vi "Transfer Images Data to UI - Copy.vi"(0 "fpga interface in":refnum<k20>, 1 "'stop' notifier":refnum<notifier>, 2 "queue out":refnum<queue>, 3 "measure call context in":refnum<class "Measure Call Context.lvclass">, 7 "display channel number":i32, 11 "error in":errorcluster, 13 "raw display notifier":refnum<notifier>) -> (4 "fpga interface out":refnum<k20>, 15 "error out":errorcluster)   [LabVIEW 2025, in "Automotive Vision.lvclass"]
doc: "Handles frame grabbing, and prepare data for sendig it to the UI."
uses:
  Automotive Vision.lvclass
  <vilib>/Plug-In SDKs/Measurements/Measure Call Context/Measure Call Context.lvclass
  <vilib>/rvi/interface/nirviReadWriteControl/nirviReadWriteControl.xnode
  Automotive Vision.lvclass/Automotive Vision.ctl
  deps/NI148X/Getting Started/Host/Common/GettingStarted_Common_148X_Host.lvlib
  deps/NI148X/Getting Started/Host/Common/Types/148x_Common_FPGA_Reference.ctl
  <instrlib>/FlexRIO/CSI-2/v2/Common/Types/LLP Data Type.ctl
  <instrlib>/FlexRIO/CSI-2/v2/Common/NI CSI-2 API Common v2.lvlib
  Automotive-Vision OOB Data Transfer/Automotive-Vision OOB Data Transfer.lvlib
  Measurement Results.ctl
  NiFpgaLv.dll
  <vilib>/Utility/error.llb/Error Cluster From Error Code.vi
  <vilib>/rvi/interface/Simulation/niFpgaSimulationCallBeginRW.vi
  <vilib>/rvi/errors/niLvFpgaAdjustHostInterfaceError.vi
  <vilib>/vision/Image Controls.llb/IMAQ Image.ctl
  deps/NI148X/Getting Started/Host/Common/Types/RAW Interpretation for Display.ctl
  deps/NI148X/Getting Started/Host/Common/Types/Serial Channel Display Parameters.ctl
  Status Data.ctl
  Image Info.ctl
panel:
  in  "Image Info":T1
  out "Image Pixels (U32)":u32[](array[numeric])
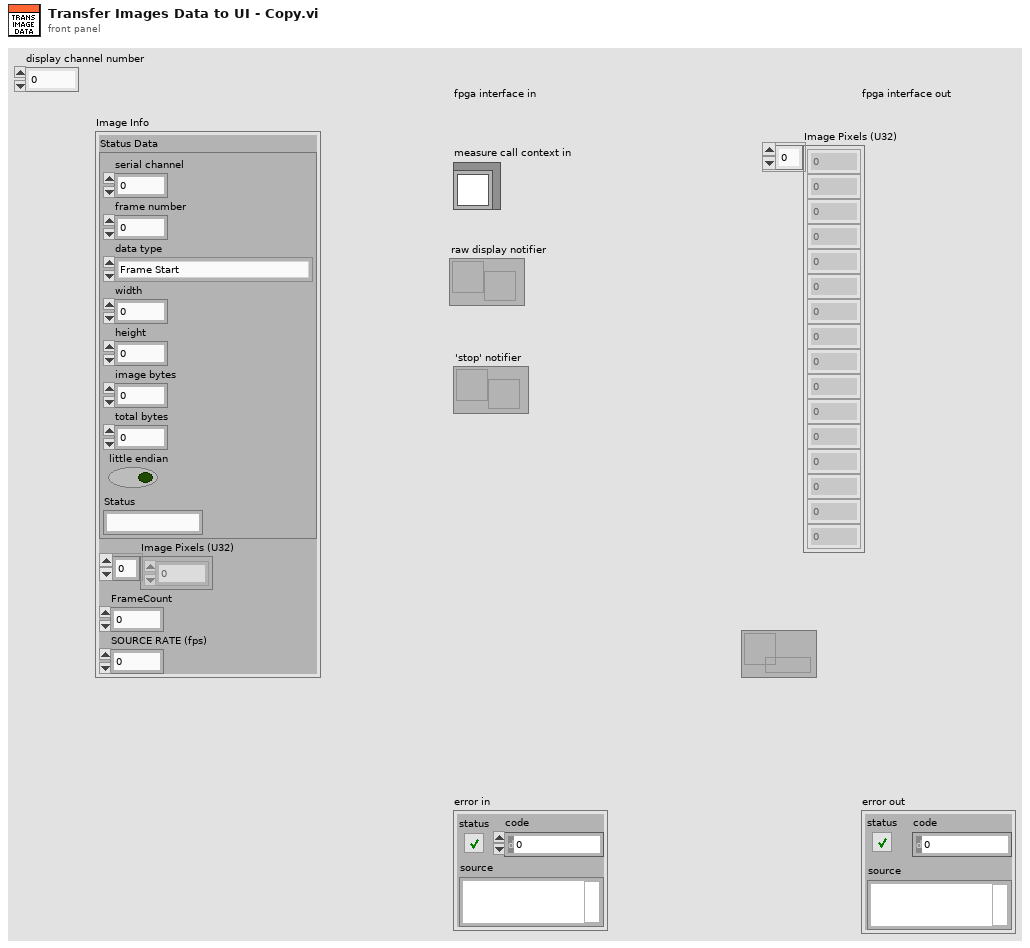
[diagram p1: front panel]
types:
  T1 = typedef "Image Info.ctl" = cluster{"Status Data":T2, "Image Pixels (U32)":u32[], "FrameCount":u64, "SOURCE RATE (fps)":dbl}
  T2 = typedef "Status Data.ctl" = cluster{"serial channel":fxp<+,3,3>, "frame number":u16, "data type":T3, "width":u16, "height":u16, "image bytes":u32, "total bytes":u32, "little endian":bool, "Status":string}
  T3 = typedef "NI CSI-2 API Common v2.lvlib/LLP Data Type.ctl" = enum8{"Frame Start", "Frame End", "Line Start", "Line End", "End of Transmission", "Reserved 0", "Reserved 1", "Reserved 2", "Generic Short Packet 1", "Generic Short Packet 2", "Generic Short Packet 3", "Generic Short Packet 4", "Generic Short Packet 5", "Generic Short Packet 6", "Generic Short Packet 7", "Generic Short Packet 8", "Null", "Blanking Data", "Embedded 8-bit non Image Data", "Generic Long Packet 1", "Generic Long Packet 2", "Generic Long Packet 3", "Generic Long Packet 4", "Reserved 3", "YUV420 8-bit", "YUV420 10-bit", "Legacy YUV420 8-bit", "Reserved 4", "YUV420 8-bit Chroma Shifted", "YUV420 10-bit Chroma Shifted", "YUV422 8-bit", "YUV422 10-bit", "RGB444", "RGB555", "RGB565", "RGB666", "RGB888", "Reserved 5", "Reserved 6", "RAW 24", "RAW 6", "RAW 7", "RAW 8", "RAW 10", "RAW 12", "RAW 14", "RAW 16", "RAW 20", "User Defined 8-bit Data 1", "User Defined 8-bit Data 2", "User Defined 8-bit Data 3", "User Defined 8-bit Data 4", "User Defined 8-bit Data 5", "User Defined 8-bit Data 6", "User Defined 8-bit Data 7", "User Defined 8-bit Data 8", "USL Command", "Reserved 7", "Reserved 8", "Reserved 9", "Reserved 10", "Reserved 11", "Reserved 12", "LRTE EPD Spacer"}
  T4 = cluster{"serial channel":fxp<+,3,3>, "frame number":u16, "data type":T3, "width":u16, "height":u16, "image bytes":u32, "total bytes":u32, "little endian":bool, "Status":string}
  T5 = typedef "GettingStarted_Common_148X_Host.lvlib/148x_Common_FPGA_Reference.ctl" = refnum<k20>
  T6 = typedef "GettingStarted_Common_148X_Host.lvlib/Serial Channel Display Parameters.ctl" = cluster{"images":cluster{"grayscale":T7, "color":T7}, "RAW parameters":cluster{"interpretation":T8, "bayer parameters":cluster{"pattern":i32, "algorithm":i32, "red gain":dbl, "green gain":dbl, "blue gain":dbl}}}
  T7 = typedef "IMAQ Image.ctl" = refnum<image>
  T8 = typedef "GettingStarted_Common_148X_Host.lvlib/RAW Interpretation for Display.ctl" = enum16{"Grayscale", "Bayer", "RGB", "YUV422", "YUV420", "Legacy YUV420"}
  T9 = typedef "GettingStarted_Common_148X_FPGA.lvlib/Image Metadata.ctl" = cluster{"serial channel":fxp<+,3,3>, "frame number":u16, "data type":T3, "width":u16, "height":u16, "image bytes":u32, "total bytes":u32, "little endian":bool}
  T10 = typedef "Automotive-Vision OOB Data Transfer.lvlib/OOB to Logic Data.ctl" = cluster{"PauseResume":bool, "ExportPath":string, "ExportType":u16, "Export":bool}
  T11 = typedef "Automotive Vision.lvclass/Measurement Results.ctl" = cluster{"ACQ. IN PROGRESS":bool, "IMAGE PIXEL DATA":u32[], "ACQ. DURATION (s)":dbl, "SOURCE RATE (fps)":dbl, "BYTES ACQUIRED":u64, "FRAME COUNT":u64, "POC VOLTAGE (V)":dbl, "POC CURRENT (A)":dbl, "ERROR":bool, "STATE MESSAGE":string, "IMAGE DATA":string, "OOB gRPC Port":i32, "HEIGHT":u64, "WIDTH":u64, "IMAGE SIZE":u64}
  T12 = cluster{"image pixel data fifo overflow":bool, "image metadata fifo overflow":bool}[]
  T13 = cluster{"image pixel data fifo overflow":bool, "image metadata fifo overflow":bool}
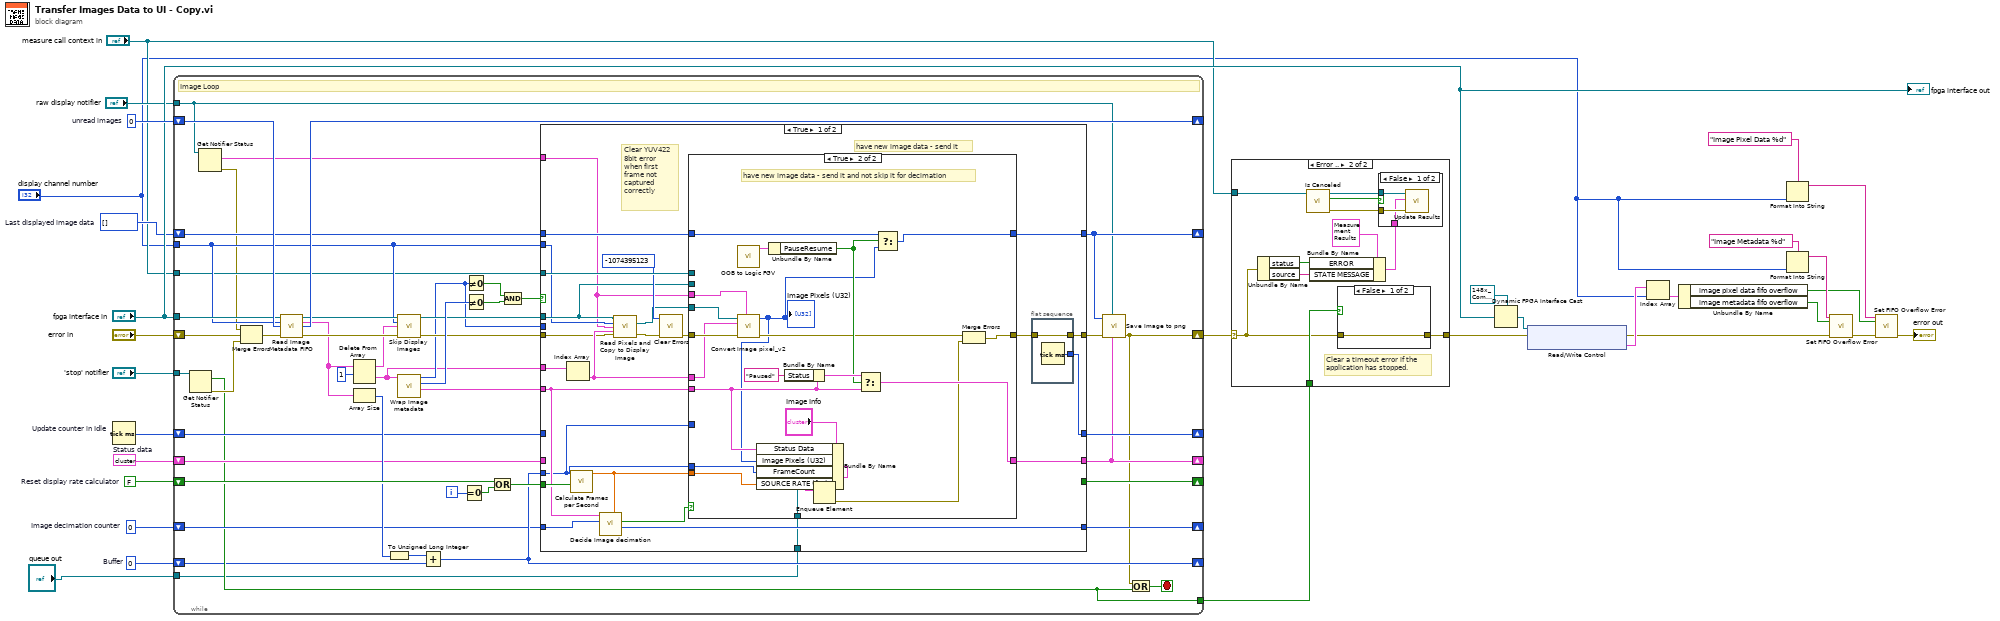
[diagram p0: block diagram]
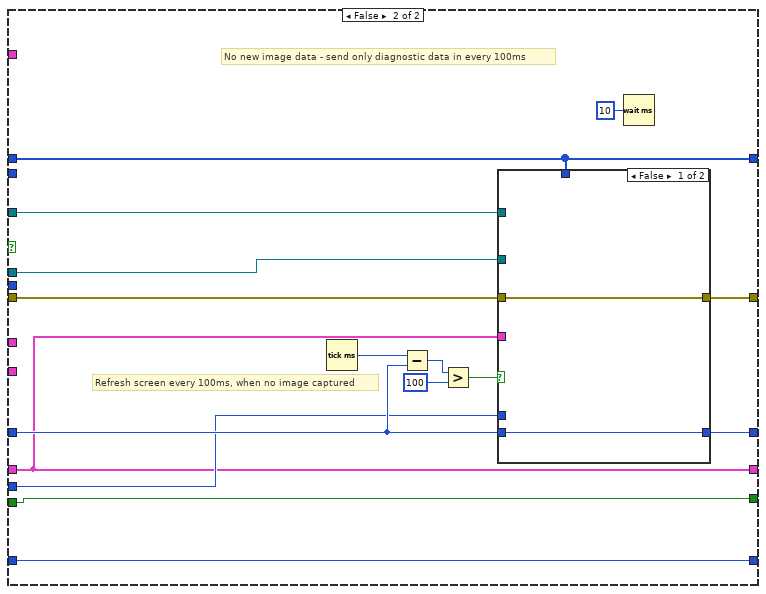
[diagram p3: hidden frame]
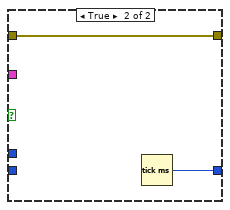
[diagram p4: hidden frame]
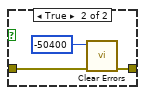
[diagram p7: hidden frame]
diagram:
  w5 = T4 {"serial channel"=0.0, "frame number"=0, "data type"=enum."Frame Start", "width"=0, "height"=0, "image bytes"=0, "total bytes"=0, "little endian"=FALSE, "Status"="Ready for Acquisition"}  # Status data
  w7 = u32 0  # Image decimation counter
  w8 = u32[] []  # Last displayed image data
  w14 = u32 0  # Buffer
  w15 = FALSE  # Reset display rate calculator
  w30 = u32 0  # unread images
  n1 = Tick Count (ms) "Update counter in Idle"() -> (millisecond timer value=w9:u32)
  n2 = while {
    shift-right: [w36] -> w13
    shift-left: "error in" -> [w53]
    tunnel: "fpga interface in" -> [w56]
    shift-right: [w76] -> _
    shift-left: w30 -> [w67]
    tunnel: "display channel number" -> [w52]
    shift-right: [w71] -> _
    shift-left: w15 -> [w68]
    shift-right: [w58] -> _
    shift-left: w14 -> [w40]
    tunnel: [w42] -> w11
    tunnel: "'stop' notifier" -> [w55]
    shift-right: [w50] -> _
    shift-left: w9 -> [w51]
    shift-right: [w39] -> _
    shift-left: w8 -> [w49]
    shift-right: [w47] -> _
    shift-left: w7 -> [w48]
    tunnel: "measure call context in" -> [w46]
    shift-right: [w37] -> _
    shift-left: w5 -> [w45]
    tunnel: "raw display notifier" -> [w35]
    tunnel: "queue out" -> [w31]
    i -> [w75]
    stop <- w77 stop-if-true
    # "Image Loop"
    n3 = Get Notifier Status(notifier=w55) -> (current notification=w42:bool, error out=w78:errorcluster)  [unwired: 1 in, 3 out]
    n4 = Get Notifier Status(notifier=w35) -> (current notification=w33:T6[], error out=w34:errorcluster)  [unwired: 1 in, 3 out]
    n5 = Merge Errors(w34, w53, w78) -> (w54:errorcluster)
    n6 = call "Read Image Metadata FIFO.vi"("fpga inteface in"=w56, "display channel number"=w52, "number of images"=w67, "error in (no error)"=w54) -> ("fpga interface out"=w64:refnum<k20>, "image metadata"=w57:T9[], "images remaining"=w76:u32, "error out"=w61:errorcluster)  [unwired: 8 in]
    n7 = Delete From Array(array=w57, length=1) -> (deleted portion=w32:T9[], array with subset deleted=w60:T9[])  [unwired: 1 in]
    n8 = Array Size(array=w57) -> (size(s)=w59:i32)
    n9 = To Unsigned Long Integer(number=w59) -> (unsigned 32bit integer=w41:u32)
    n10 = call "Skip Display Images.vi"("fpga interface in"=w64, "display channel number"=w52, "image metadata"=w60, "error in (no error)"=w61) -> ("fpga interface out"=w63:refnum<k20>, "error out"=w62:errorcluster)  [unwired: 10 in]
    n11 = call "Wrap Image metadata.vi"("image metadata"=w32) -> ("element"=w44:T4, "Numeric"=w66:i32, "total bytes"=w43:u32)  [unwired: 8 in]
    n12 = Add(x=w41, y=w40) -> (x+y=w58:u32)
    n13 = Equal To 0?(x=w75) -> (x = 0?=w69:bool)
    n14 = Not Equal To 0?(x=w43) -> (x != 0?=w73:bool)
    n15 = Not Equal To 0?(x=w66) -> (x != 0?=w74:bool)
    n16 = Compound Arithmetic op=OR(w68, w69) -> (w70:bool)
    n17 = Compound Arithmetic op=AND(w73, w74) -> (w72:bool)
    n18 = case shown="True" w72 {
      tunnel: w62 -> [w81 w130]
      tunnel: w63 -> [w85 w129]
      tunnel: w52 -> [w84 _]
      tunnel: [w101 w137] -> w38
      tunnel: w70 -> [w93 w144]
      tunnel: [_ w144] -> w71
      tunnel: w58 -> [w79 w134]
      tunnel: w43 -> [_ _]
      tunnel: w44 -> [w90 _]
      tunnel: w46 -> [w102 w131]
      tunnel: w51 -> [_ w136]
      tunnel: [w100 w138] -> w50
      tunnel: w49 -> [w98 w135]
      tunnel: [w99 w135] -> w39
      tunnel: w48 -> [w97 w133]
      tunnel: [w96 w133] -> w47
      tunnel: w45 -> [_ w132]
      tunnel: [w94 w132] -> w37
      tunnel: w33 -> [w83 _]
      tunnel: w32 -> [w91 _]
      tunnel: w31 -> [w80 _]
      frame True {
        # "Clear YUV422 8bit error when first frame not captured correctly"
        # "have new image data - send it"
        n19 = Index Array(array=w91) -> (element=w82:T9)  [unwired: 1 in]
        n20 = call <vilib>:"Calculate Frames per Second.vi"("Reset"=w93, "Buffer Number"=w79) -> ("Acquired Frames/s"=w89:dbl)  [unwired: 7 in, 2 out]
        n21 = call "Decide Image decimation.vi"("FPS"=w89, "Image decimation counter in"=w97, "element in"=w90) -> ("Image decimation counter out"=w96:u32, "send current image data"=w95:bool)  [unwired: 7 in]
        n22 = call "Read Pixels and Copy to Display Image.vi"("fpga interface in"=w85, "display channel number"=w84, "serial channel display parameters"=w83, "image metadata"=w82) -> ("display image"=w86:T7)  [unwired: 9 in, 2 out]
        n23 = call <vilib>:"Clear Errors.vi"("error in (no error)"=w81, "specific error code to clear (0: all)"=-1074395123) -> ("error out"=w87:errorcluster)  [unwired: 4 in, 1 out]
        n24 = case shown="True" w95 {
          tunnel: [w103 w113] -> w92
          tunnel: w89 -> [_ w106]
          tunnel: w90 -> [w104 w110]
          tunnel: w102 -> [_ _]
          tunnel: [w105 w126] -> w99
          tunnel: w79 -> [_ _]
          tunnel: w98 -> [w105 w125]
          tunnel: [w104 w124] -> w94
          tunnel: w85 -> [_ _]
          tunnel: w87 -> [w103 w119]
          tunnel: w86 -> [_ w117]
          tunnel: w82 -> [_ w116]
          tunnel: w83 -> [_ w115]
          tunnel: w80 -> [_ w114]
          tunnel: w79 -> [_ w107]
          frame False {
            # "have new image data - but skip the sending to not overload UI with data transfer"
          }
          frame True {
            # "have new image data - send it and not skip it for decimation"
            n25 = call "OOB to Logic FGV.vi"() -> ("OOB to Logic Data out"=w121:T10)  [unwired: 10 in, 1 out]
            n26 = call "Convert Image pixel_v2.vi"("serial channel display parameters"=w115, "error in"=w119, "image metadata"=w116, "Refnum in"=w117) -> ("error out"=w118:errorcluster, "Image Pixels (U32)"=w109:u32[])  [unwired: 6 in]
            "Image Pixels (U32)" <- w109
            n27 = Bundle By Name(cluster="Image Info", "Status Data"=w110, "Image Pixels (U32)"=w109, "FrameCount"=w107, "SOURCE RATE (fps)"=w106) -> (w108:T1)
            n28 = Unbundle By Name(w121) -> ("PauseResume"=w120:bool)
            n29 = Bundle By Name(cluster=w110, "Status"="Paused") -> (w123:T4)
            n30 = Enqueue Element(queue=w114, element=w108) -> (error out=w112:errorcluster)  [unwired: 2 in, 2 out]
            n31 = Select(t=w123, s=w120, f=w110) -> (s? t:f=w124:T4)
            n32 = Select(t=w125, s=w120, f=w109) -> (s? t:f=w126:u32[])
            n33 = Merge Errors(w118, w112) -> (w113:errorcluster)
          }
        }
        n34 = flat-sequence {
          tunnel: [w128] -> w101
          tunnel: w92 -> [w128]
          tunnel: [w127] -> w100
          frame #0 {
            n35 = Tick Count (ms)() -> (millisecond timer value=w127:u32)
          }
        }
      }
      frame False {
        # "Refresh screen every 100ms, when no image captured"
        # "No new image data - send only diagnostic data in every 100ms"
        n36 = Tick Count (ms)() -> (millisecond timer value=w142:u32)
        n37 = Subtract(x=w142, y=w136) -> (x-y=w141:u32)
        n38 = Greater?(x=w141, y=u32 100) -> (0:w139:bool)
        n39 = case shown="False" w139 {
          tunnel: w130 -> [w146 w147]
          tunnel: [w146 w147] -> w137
          tunnel: w132 -> [_ _]
          tunnel: [w145 w148] -> w138
          tunnel: w136 -> [w145 _]
          tunnel: w135 -> [_ _]
          tunnel: w134 -> [_ _]
          tunnel: w131 -> [_ _]
          tunnel: w129 -> [_ _]
          frame False {
          }
          frame True {
            n40 = Tick Count (ms)() -> (millisecond timer value=w148:u32)
          }
        }
        n41 = Wait (ms)(milliseconds to wait=u32 10) -> ()  [unwired: 1 out]
      }
    }
    n42 = call "Save Image to png.vi"("image metadata"=w37, "raw display notifier"=w35, "error in"=w38, "Last displayed image data"=w39) -> ("error out"=w36:errorcluster)  [unwired: 7 in]
    n43 = Compound Arithmetic op=OR(w36, w42) -> (w77:bool)
  }
  n44 = case shown="Error .." w13 {
    selector: w13 -> [w149 w153]
    tunnel: [w149 w160] -> w25
    tunnel: w11 -> [_ w159]
    tunnel: "measure call context in" -> [_ w150]
    frame No Error {
    }
    frame Error {
      # "Clear a timeout error if the application has stopped."
      n45 = Unbundle By Name(w153) -> ("status"=w152:bool, "source"=w151:string)
      n46 = call <vilib>:"Is Canceled.vi"("measure call context in"=w150) -> ("error out"=w157:errorcluster, "is canceled?"=w156:bool, "measure call context out"=w158:refnum<class "Measure Call Context.lvclass">)  [unwired: 8 in]
      n47 = Bundle By Name(cluster=T11 {"ACQ. IN PROGRESS"=FALSE, "IMAGE PIXEL DATA"=[], "ACQ. DURATION (s)"=0.0, "SOURCE RATE (fps)"=0.0, "BYTES ACQUIRED"=0, "FRAME COUNT"=0, "POC VOLTAGE (V)"=0.0, "POC CURRENT (A)"=0.0, "ERROR"=FALSE, "STATE MESSAGE"="", "IMAGE DATA"="", "OOB gRPC Port"=0, "HEIGHT"=0, "WIDTH"=0, "IMAGE SIZE"=0} ("Measurement Results"), "ERROR"=w152, "STATE MESSAGE"=w151) -> (w154:T11)
      n48 = case shown="False" w159 {
        tunnel: w153 -> [w164 w167]
        tunnel: [w164 w165] -> w160
        frame False {
        }
        frame True {
          n49 = call <vilib>:"Clear Errors.vi"("error in (no error)"=w167, "specific error code to clear (0: all)"=-50400 ("y")) -> ("error out"=w165:errorcluster)  [unwired: 4 in, 1 out]
        }
      }
      n50 = case shown="False" w156 {
        tunnel: w158 -> [w163 _]
        tunnel: w157 -> [w162 _]
        tunnel: w154 -> [w161 _]
        frame False {
          n51 = call <vilib>:"Update Results.vi"("error in"=w162, "measurement results"=w161, "measure call context in"=w163) -> ()  [unwired: 7 in, 2 out]
        }
        frame True {
        }
      }
    }
  }
  n52 = Dynamic FPGA Interface Cast(Session In=T5 refnum ("FPGA VI Reference Out"), Type="fpga interface in") -> (Session Out=w26:T5)
  n53 = xnode ("Read/Write Control")("FPGA VI Reference In"=w26, "error in"=w25) -> ("error out"=w24:errorcluster, "display channel status"=w28:T12)  [unwired: 1 out]
  n54 = Index Array(array=w28, index="display channel number") -> (element=w29:T13)
  n55 = Unbundle By Name(w29) -> ("image pixel data fifo overflow"=w17:bool, "image metadata fifo overflow"=w16:bool)
  n56 = Format Into String(format string="Image Pixel Data %d", "display channel number") -> (resulting string=w19:string)  [unwired: 2 in, 1 out]
  n57 = Format Into String(format string="Image Metadata %d", "display channel number") -> (resulting string=w18:string)  [unwired: 2 in, 1 out]
  n58 = call "Set FIFO Overflow Error.vi"("fifo name"=w18, "overflow"=w16, "error in (no error)"=w24) -> ("error out"=w21:errorcluster)  [unwired: 12 in]
  n59 = call "Set FIFO Overflow Error.vi"("fifo name"=w19, "overflow"=w17, "error in (no error)"=w21) -> ("error out"=→"error out":errorcluster)  [unwired: 12 in]
  "fpga interface out" <- "fpga interface in"
